vi "Constant_FilePaths.vi"() -> (2 "Paths":T1)   [LabVIEW 2016]
uses:
  Constant_FilePaths_ctl.ctl
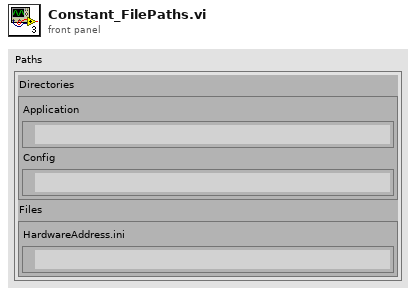
[diagram p1: front panel]
types:
  T1 = typedef "Constant_FilePaths_ctl.ctl" = cluster{"Directories":cluster{"Application":path, "Config":path}, "Files":cluster{"HardwareAddress.ini":path}}
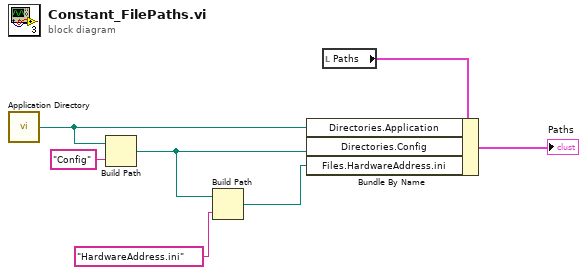
[diagram p0: block diagram]
diagram:
  n1 = call <vilib>:"Application Directory.vi"() -> ("Application Directory"=w4:path)
  n2 = Build Path(base path=w4, name or relative path="Config") -> (appended path=w3:path)
  n3 = Build Path(base path=w3, name or relative path="HardwareAddress.ini") -> (appended path=w2:path)
  n4 = local read "Paths"() -> (w5:T1)
  n5 = Bundle By Name(cluster=w5, "Directories.Application"=w4, "Directories.Config"=w3, "Files.HardwareAddress.ini"=w2) -> (→"Paths":T1)
